vi "SH_readData.vi"(8 "error in (no error)":errorcluster, 9 "ControlRefs":T2, 10 "NumberOfChannels":i32, 11 "Data File":path) -> (0 "error out":errorcluster, 2 "CLassLabels out":string[](array[string]), 3 "ArrayOfTrials":T1(array[cluster]))   [LabVIEW 2016, in "Shapelets Search (Brute Force).lvlib"]
uses:
  Shapelets Search (Brute Force).lvlib
  <vilib>/xml/Load XML File.vi
  <vilib>/xml/Close Reference(Node).vi
  _XML_EEG_Features/XML_EEG_Features.lvlib
  <vilib>/xml/NI_XML.lvlib
panel:
  # "This VI is a part of BCI Design library, http://www.ru-bci.org \nCopyright © 2020, Sotnikov Peter, All rights reserved. License: CC BY-NC 4.0"
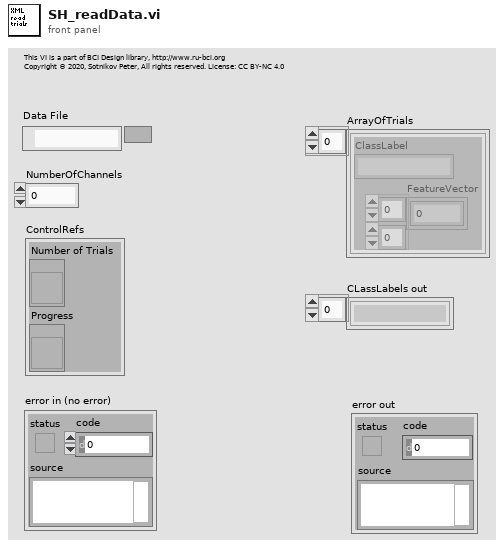
[diagram p1: front panel]
types:
  T1 = cluster{"ClassLabel":string, "FeatureVector":dbl[][]}[]
  T2 = cluster{"Number of Trials":refnum<vi>, "Progress":refnum<vi>}
  T3 = typedef "XML_EEG_Features.lvlib/XML_FF_Header.ctl" = cluster{"NumberOfTrials":i32, "NumberOfClasses":i32, "FeatureVectorLength":i32, "FeatureExtractionMethod":string}
  T4 = typedef "XML_EEG_Features.lvlib/XML_FF_Trial.ctl" = cluster{"ClassLabel":string, "FeatureVector":dbl[]}
  T5 = cluster{"ClassLabel":string, "FeatureVector":dbl[][]}
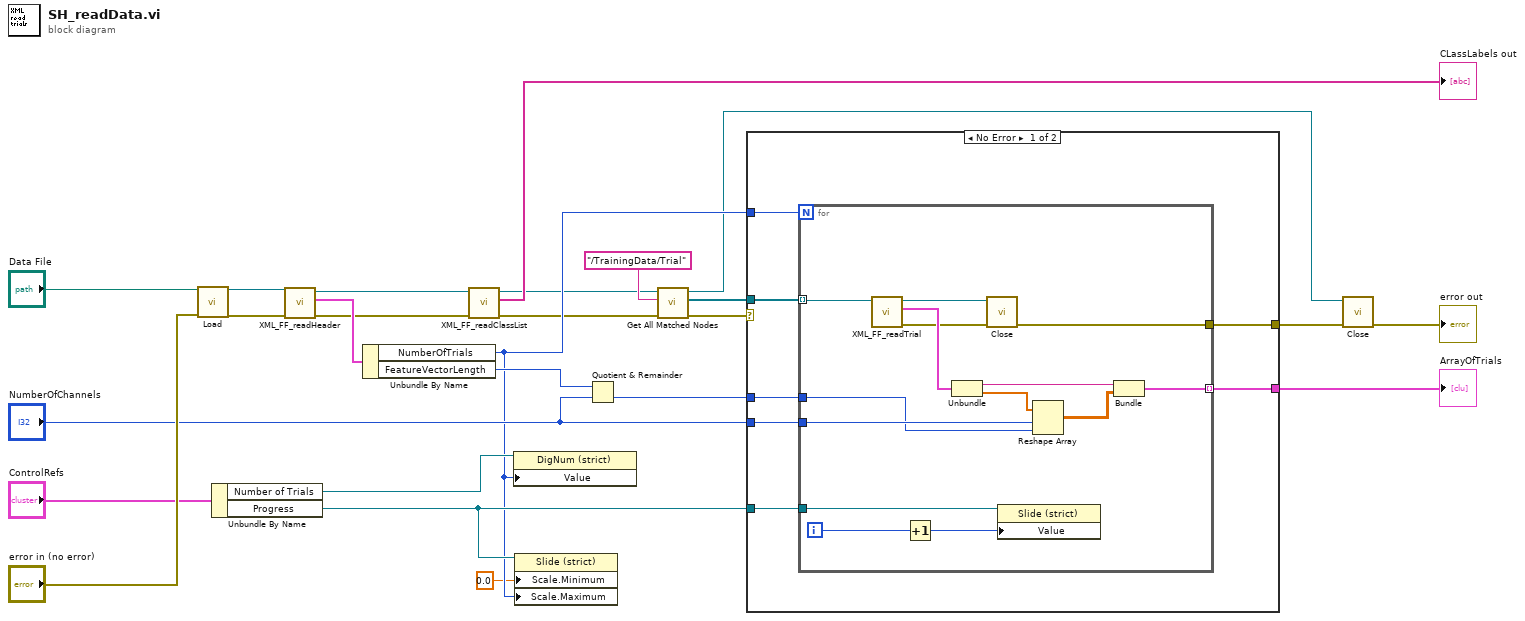
[diagram p0: block diagram]
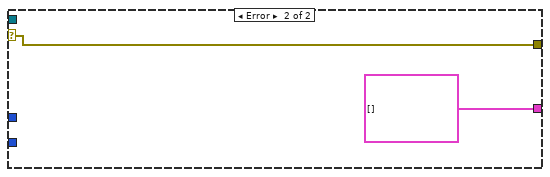
[diagram p2: hidden frame]
diagram:
  n1 = call-poly <vilib>:"Load.vi"("path to XML document"="Data File", "error in (no error)"="error in (no error)") -> ("DOM document out"=w23:refnum<k20>, "error out"=w22:errorcluster)  [unwired: 11 in, 1 out]
  n2 = Unbundle By Name("ControlRefs") -> ("Number of Trials"=w15:refnum<vi>, "Progress"=w14:refnum<vi>)
  n3 = call "XML_FF_readHeader.vi"("error in (no error)"=w22, "DOM document in"=w23) -> ("error out"=w8:errorcluster, "FF_Header out"=w21:T3, "DOM document out"=w9:refnum<k20>)  [unwired: 7 in]
  n4 = Unbundle By Name(w21) -> ("NumberOfTrials"=w13:i32, "FeatureVectorLength"=w19:i32)
  n5 = call "XML_FF_readClassList.vi"("error in (no error)"=w8, "DOM document in"=w9) -> ("error out"=w4:errorcluster, "CLassLabels out"=→"CLassLabels out":string[], "DOM document out"=w5:refnum<k20>)  [unwired: 7 in]
  n6 = property class="DigNum (strict)"(reference=w15, "Value"=w13) -> ()  [unwired: 1 in, 2 out]
  n7 = property class="Slide (strict)"(reference=w14, "Scale.Minimum"=0.0 ("Scale.Range:Minimum"), "Scale.Maximum"=w13) -> ()  [unwired: 1 in, 2 out]
  n8 = Quotient & Remainder(x=w19, y="NumberOfChannels") -> (floor(x/y)=w17:i32)  [unwired: 1 out]
  n9 = call <vilib>:"Get All Matched Nodes.vi"("error in (no error)"=w4, "XPath expression"="/TrainingData/Trial", "node in"=w5) -> ("error out"=w2:errorcluster, "node result array"=w3:refnum<k20>[], "node out"=w1:refnum<k20>)  [unwired: 6 in]
  n10 = case shown="No Error" w2 {
    selector: w2 -> [_ w47]
    tunnel: w13 -> [w32 _]
    tunnel: "NumberOfChannels" -> [w31 _]
    tunnel: w17 -> [w30 _]
    tunnel: [w29 T1 []] -> w16
    tunnel: w14 -> [w28 _]
    tunnel: [w27 w47] -> w10
    tunnel: w3 -> [w26 _]
    frame No Error {
      n11 = for {
        N: w32 -> [_]
        tunnel: w26 -> [w46] mode=indexing
        tunnel: w31 -> [w43]
        tunnel: w30 -> [w42]
        tunnel: [w39] -> w29 mode=indexing
        tunnel: w28 -> [w38]
        tunnel: [w35] -> w27
        i -> [w34]
        n12 = call "XML_FF_readTrial.vi"("DOM document in"=w46) -> ("error out"=w36:errorcluster, "Trial out"=w45:T4, "DOM document out"=w37:refnum<k20>)  [unwired: 8 in]
        n13 = Increment(x=w34) -> (x+1=w33:i32)
        n14 = Unbundle(w45) -> ("ClassLabel"=w41:string, "FeatureVector"=w44:dbl[])
        n15 = call-poly <vilib>:"Close.vi"("error in (no error)"=w36, "node"=w37) -> ("error out"=w35:errorcluster)  [unwired: 7 in]
        n16 = property class="Slide (strict)"(reference=w38, "Value"=w33) -> ()  [unwired: 1 in, 2 out]
        n17 = Reshape Array(w44, w43, w42) -> (w40:dbl[][])
        n18 = Bundle("ClassLabel"=w41, "FeatureVector"=w40) -> (w39:T5)  [unwired: 1 in]
      }
    }
    frame Error {
    }
  }
  "ArrayOfTrials" <- w16
  n19 = call-poly <vilib>:"Close.vi"("error in (no error)"=w10, "node"=w1) -> ("error out"=→"error out":errorcluster)  [unwired: 7 in]
